vi "adam-write-&-check-response.vi"(8 "error in (no error)":errorcluster, 10 "write buffer":string, 11 "VISA resource name":refnum<visa-resource-name>) -> (0 "error out":errorcluster, 1 "cmd aknowledged":bool, 2 "acknowledge char":string, 3 "VISA resource name out":refnum<visa-resource-name>, 4 "read buffer":string, 5 "read return":u32)   [LabVIEW 2024]
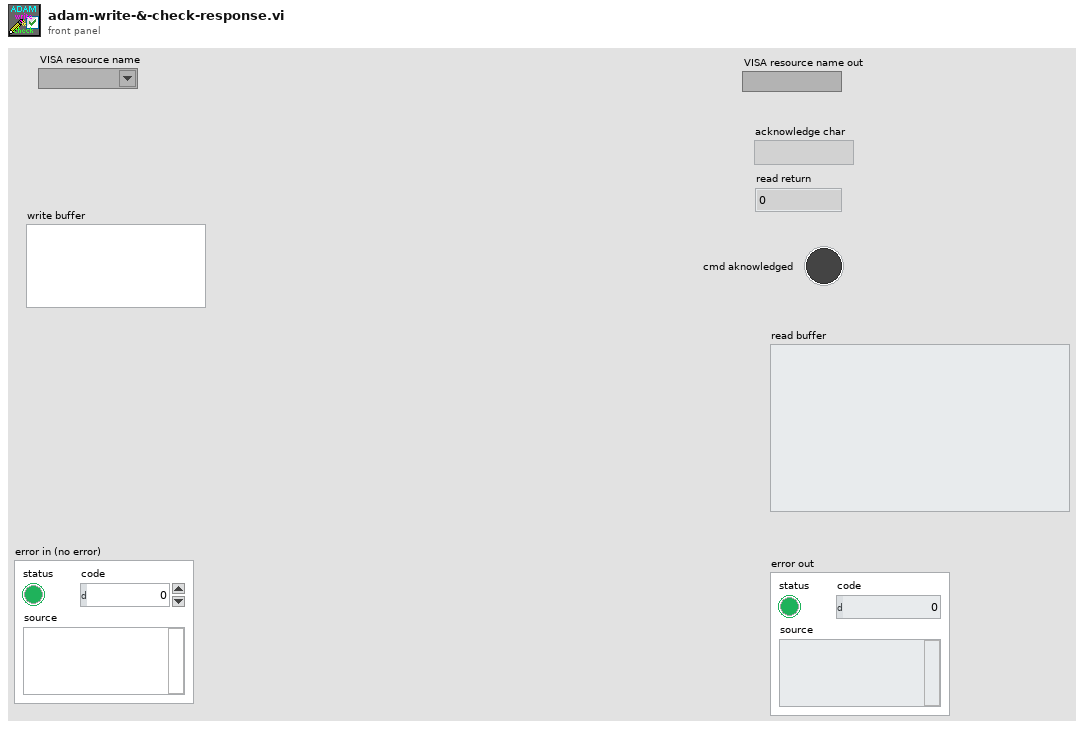
[diagram p1: front panel]
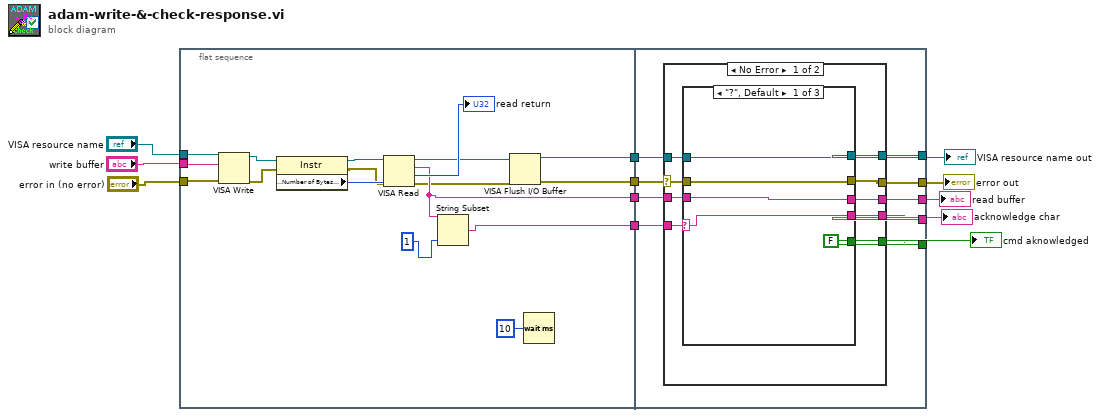
[diagram p0: block diagram]
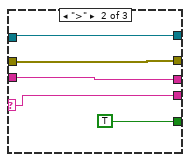
[diagram p2: hidden frame]
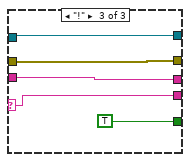
[diagram p3: hidden frame]
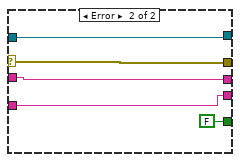
[diagram p4: hidden frame]
diagram:
  n1 = flat-sequence {
    tunnel: "write buffer" -> [w16]
    tunnel: "VISA resource name" -> [w15]
    tunnel: "error in (no error)" -> [w14]
    tunnel: [w22] -> w9
    tunnel: [w21] -> w8
    tunnel: [w18] -> w7
    tunnel: [w17] -> w6
    tunnel: w9 -> [w37]
    tunnel: w8 -> [w35]
    tunnel: w7 -> [w38]
    tunnel: w6 -> [w36]
    tunnel: [w34] -> w5
    tunnel: [w33] -> w4
    tunnel: [w32] -> w3
    tunnel: [w31] -> w2
    tunnel: [w30] -> w1
    frame #0 {
      n2 = VISA Write(VISA resource name=w15, write buffer=w16, error in (no error)=w14) -> (VISA resource name out=w24:refnum<visa-resource-name>, error out=w23:errorcluster)  [unwired: 1 out]
      n3 = property class="Instr"(reference=w24, error in=w23) -> (reference out=w27:refnum<visa-resource-name>, error out=w28:errorcluster, "Serial Settings:Number of Bytes at Serial Port"=w29:u32)
      n4 = VISA Read(VISA resource name=w27, byte count=w29, error in (no error)=w28) -> (VISA resource name out=w20:refnum<visa-resource-name>, read buffer=w21:string, return count=→"read return":u32, error out=w19:errorcluster)
      n5 = String Subset(string=w21, length (rest)=1 ("length (rest)")) -> (substring=w22:string)  [unwired: 1 in]
      n6 = VISA Flush I/O Buffer(VISA resource name=w20, error in (no error)=w19) -> (VISA resource name out=w17:refnum<visa-resource-name>, error out=w18:errorcluster)  [unwired: 1 in]
      n7 = Wait (ms)(milliseconds to wait=u32 10) -> ()  [unwired: 1 out]
    }
    frame #1 {
      n8 = case shown="No Error" w38 {
        selector: w38 -> [w43 w67]
        tunnel: [w47 FALSE ("cmd aknowledged")] -> w34
        tunnel: w37 -> [w46 w66]
        tunnel: [w45 w66] -> w33
        tunnel: [w44 w67] -> w32
        tunnel: w36 -> [w42 w64]
        tunnel: [w41 w64] -> w31
        tunnel: [w40 w63] -> w30
        tunnel: w35 -> [w39 w63]
        frame No Error {
          n9 = case shown="\"?\", Default" w46 {
            selector: w46 -> [w51 w56 w61]
            tunnel: [FALSE ("cmd aknowledged") TRUE ("cmd aknowledged") TRUE ("cmd aknowledged")] -> w47
            tunnel: [w51 w56 w61] -> w45
            tunnel: [w50 w55 w60] -> w44
            tunnel: w43 -> [w50 w55 w60]
            tunnel: w42 -> [w49 w54 w59]
            tunnel: [w49 w54 w59] -> w41
            tunnel: [w48 w53 w58] -> w40
            tunnel: w39 -> [w48 w53 w58]
            frame "?", Default {
            }
            frame ">" {
            }
            frame "!" {
            }
          }
        }
        frame Error {
        }
      }
    }
  }
  "error out" <- w3
  "VISA resource name out" <- w2
  "cmd aknowledged" <- w5
  "acknowledge char" <- w4
  "read buffer" <- w1
